vi "多路分流器测试.vi"() -> ()   [LabVIEW 2021]
uses:
  <vilib>/Utility/file.llb/Read Delimited Spreadsheet (DBL).vi
  <vilib>/Utility/file.llb/Write Delimited Spreadsheet (string).vi
  <instrlib>/Keithley 27XX/Keithley 27XX.lvlib
  <instrlib>/TDK-Lambda G Series/TDK-Lambda G Series.lvlib
  <instrlib>/Keithley DMM6500 DAQ6500 Series/Keithley DMM6500 DAQ6500 Series.lvlib
panel:
  out "报文数组":string[][](array[string])
  out "10帧平均总判定":bool
  out "判定 2":bool[](array[boolean])
  out "10帧平均误差":dbl[](array[numeric])
  in  "传感器缩放系数":dbl=2000.0 format="%#_13g"
  in  "产品类型":string
  in  "零漂2":dbl=0.01 format="%#_13g"
  in  "精度":dbl=0.005 format="%#_13g"
  out "误差":dbl[](array[numeric])
  out "解析电流":dbl[](array[numeric])
  out "判定":bool
  out "判定":bool[](array[boolean])
  in  "CAN卡类型选择":T1
  in  "ID":string
  in  "CAN通道in":u16[](array[numeric])=[81, 82, 83]
  in  "file path (dialog if empty)":path caption="文件路径 （空时为对话框）"
  out "延迟时间":dbl[](array[numeric])=[0.0, 20.0, 5.0, 5.0, 1.0, 0.1, 0.1, 0.1, 0.1, 0.1, 0.1]
  in  "2700":refnum<visa-resource-name>="GPIB0::16::INSTR"
  out "测试电流":dbl[](array[numeric])=[0.0, 50.0, 100.0, 150.0, 200.0, 250.0, 300.0, 350.0, 400.0, 500.0, 1000.0]
  out "实际电流":dbl[](array[numeric])
  # "数据文件在F:\\shunt"
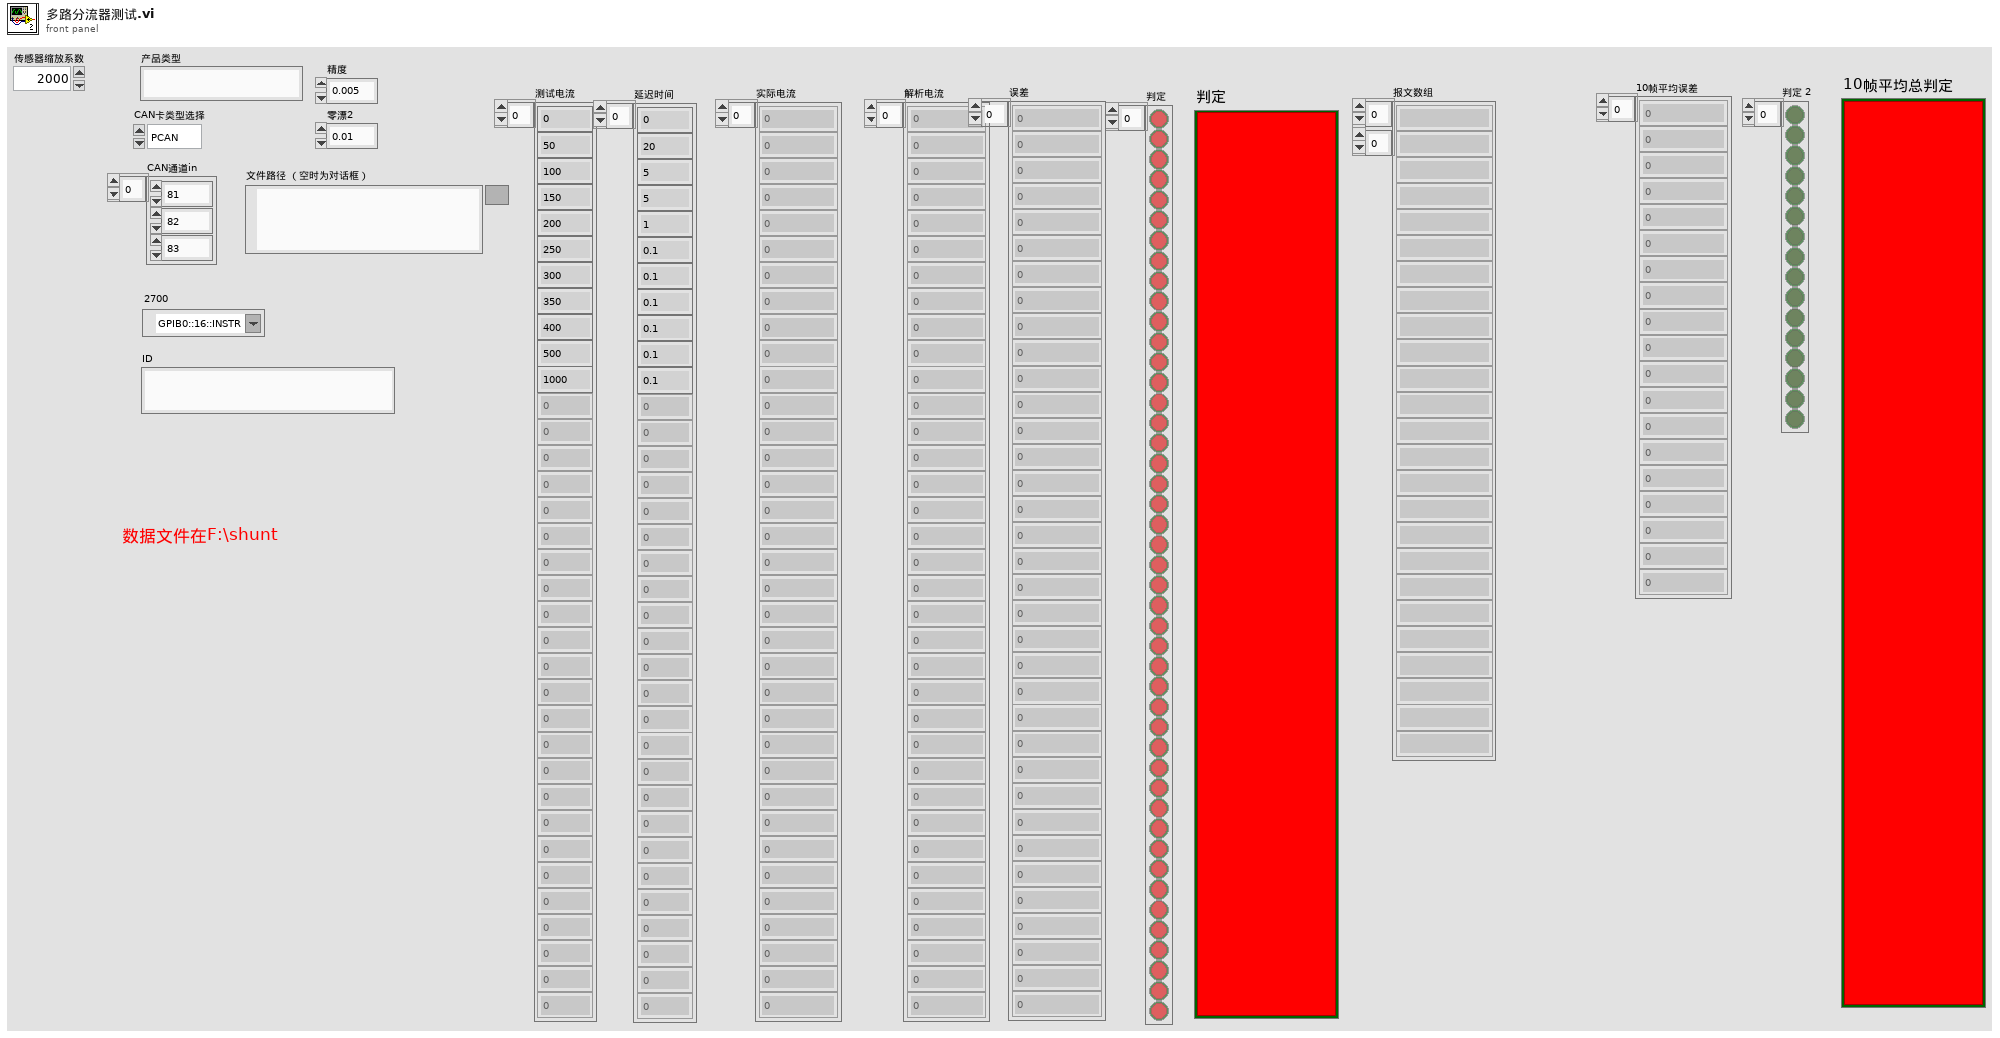
[diagram p1: front panel]
types:
  T1 = typedef "CAN type.ctl" = enum16{"PCAN", "PCANFD"}
  T2 = enum16{"open", "replace", "create", "open or create", "replace or create", "replace or create with confirmation"}
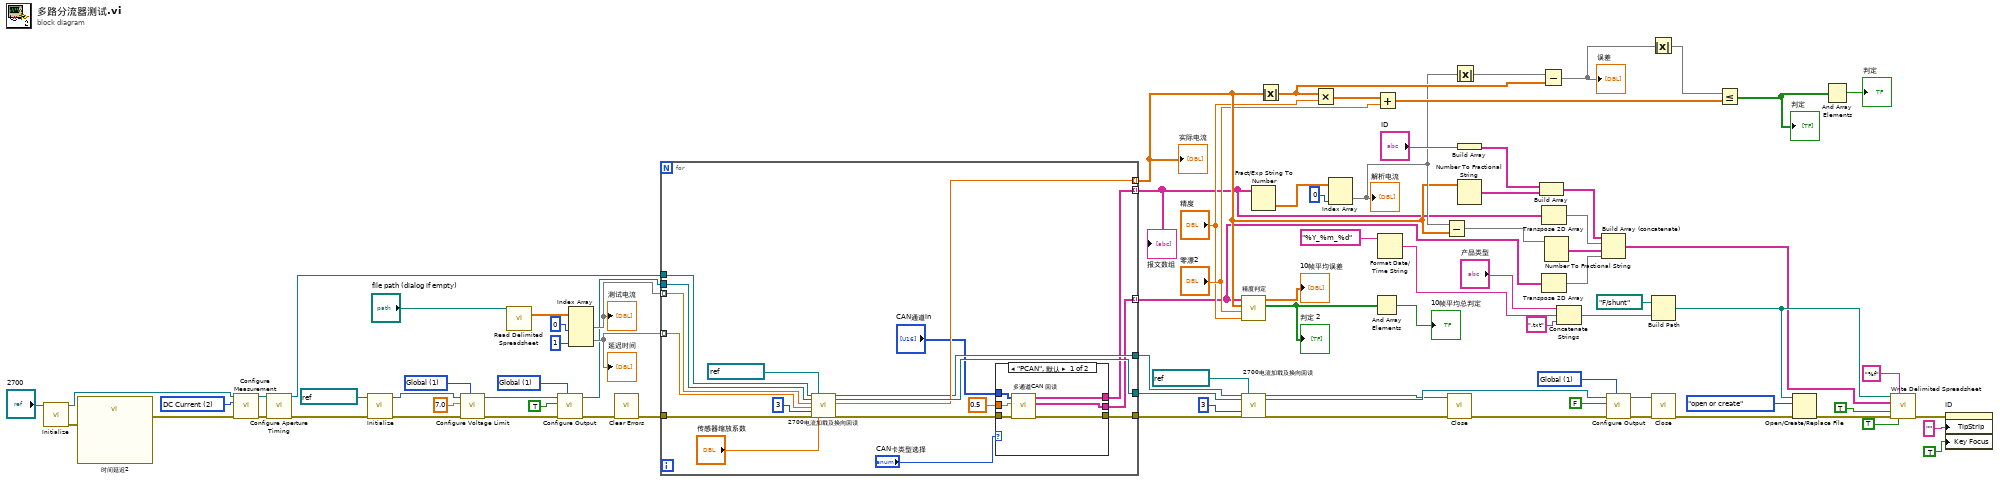
[diagram p0: block diagram]
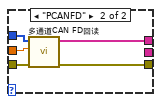
[diagram p2: hidden frame]
diagram:
  w39 = u16 2 items=["DC Voltage", "AC Voltage", "DC Current", "AC Current", "Resistance", "Four-Wire Resistance", "Temperature", "Frequency", "Period", "Continuity"] ("Function (0: DC Voltage)")
  w72 = u16 1 items=["Single", "Global"] ("Globalize (0: Single)")
  w74 = u16 1 items=["Single", "Global"] ("Globalize (0: Single)")
  w78 = u16 1 items=["Single", "Global"] ("Globalize (0: Single)")
  n1 = call <instrlib>:"Initialize.vi"("VISA resource name"="2700") -> ("VISA resource name out"=w41:refnum<visa-resource-name>, "error out"=w42:errorcluster)  [unwired: 13 in]
  n2 = call "时间延迟2"("error in (no error)"=w42) -> ("error out"=w40:errorcluster)  [unwired: 10 in]
  n3 = call <instrlib>:"Configure Measurement.vi"("VISA resource name"=w41, "Function (0: DC Voltage)"=w39, "error in (no error)"=w40) -> ("VISA resource name out"=w38:refnum<visa-resource-name>, "error out"=w37:errorcluster)  [unwired: 11 in]
  n4 = call <instrlib>:"Configure Aperture Timing.vi"("VISA resource name"=w38, "error in (no error)"=w37) -> ("VISA resource name out"=w32:refnum<visa-resource-name>, "error out"=w36:errorcluster)  [unwired: 12 in]
  n5 = call <instrlib>:"Initialize.vi"("error in (no error)"=w36, "VISA resource name"=refnum<visa-resource-name> "COM15") -> ("error out"=w79:errorcluster, "VISA resource name out"=w80:refnum<visa-resource-name>)  [unwired: 8 in]
  n6 = call <instrlib>:"Configure Voltage Limit.vi"("Globalize (0: Single)"=w78, "error in (no error)"=w79, "Voltage Limit (0V)"=7.0, "VISA resource name"=w80) -> ("error out"=w77:errorcluster, "VISA resource name out"=w76:refnum<visa-resource-name>)  [unwired: 6 in]
  n7 = call-poly <vilib>:"Read Delimited Spreadsheet.vi"("file path (dialog if empty)"="file path (dialog if empty)") -> ("all rows"=w55:dbl[][])  [unwired: 9 in, 5 out]
  n8 = call <instrlib>:"Configure Output.vi"("Globalize (0: Single)"=w74, "error in (no error)"=w77, "Enable Output (False)"=TRUE, "VISA resource name"=w76) -> ("error out"=w35:errorcluster, "VISA resource name out"=w33:refnum<visa-resource-name>)  [unwired: 6 in]
  n9 = Index Array(array=w55, index (col) #1=0 ("禁用的索引 (列)"), index (col) #2=1 ("索引 (列)")) -> (element #1=w52:dbl[], element #2=w51:dbl[])  [unwired: 2 in]
  "测试电流" <- w52
  "延迟时间" <- w51
  n10 = call <vilib>:"Clear Errors.vi"("error in (no error)"=w35) -> ("error out"=w34:errorcluster)  [unwired: 5 in, 1 out]
  n11 = for {
    tunnel: w33 -> [w94]
    tunnel: w34 -> [w102]
    tunnel: [w100] -> w83
    tunnel: [w88] -> w46
    tunnel: [w99] -> w8 mode=indexing
    tunnel: w52 -> [w98] mode=indexing
    tunnel: w51 -> [w96] mode=indexing
    tunnel: w32 -> [w95]
    tunnel: [w93] -> w50
    tunnel: [w87] -> w1 mode=indexing
    tunnel: [w85] -> w2 mode=indexing
    n12 = call "2700电流加载及换向回读.vi"("6510 in"=w95, "TDK in"=w94, "输入电流"=w98, "Delay Time (s)"=w96, "电源台数"=u8 3, "error in"=w102, "modbusin"=refnum<visa-resource-name> "COM12" ("VISA resource name"), "y"="传感器缩放系数") -> ("2700 out"=w93:refnum<visa-resource-name>, "TDK out"=w100:refnum<visa-resource-name>, "实际电流"=w99:dbl, "error out"=w91:errorcluster)  [unwired: 8 in]
    n13 = case shown="\"PCAN\", 默认" "CAN卡类型选择" {
      tunnel: w91 -> [w108 w111]
      tunnel: 0.5 ("Delay Time (s)") -> [w107 w112]
      tunnel: "CAN通道in" -> [w106 w113]
      tunnel: [w105 w110] -> w88
      tunnel: [w103 w109] -> w87
      tunnel: [w104 _] -> w85
      frame "PCAN", Default {
        n14 = call "多通道CAN 回读.vi"("错误输入（无错误）"=w108, "Delay Time (s)"=w107, "CAN通道in"=w106) -> ("错误输出"=w105:errorcluster, "10次平均"=w104:string[], "报文数组"=w103:string[])  [unwired: 6 in]
      }
      frame "PCANFD" {
        n15 = call "多通道CAN FD回读.vi"("错误输入（无错误）"=w111, "Delay Time (s)"=w112, "CAN通道in"=w113) -> ("错误输出"=w110:errorcluster, "报文数组"=w109:string[])  [unwired: 7 in]
      }
    }
  }
  "实际电流" <- w8
  "报文数组" <- w1
  n16 = call "精度判定.vi"("精度"="精度", "零飘"="零漂2", "实际电流"=w8, "报文数组"=w2) -> ("判定"=w3:bool[], "误差"=→"10帧平均误差":dbl[])  [unwired: 6 in]
  "判定 2" <- w3
  n17 = call "2700电流加载及换向回读.vi"("6510 in"=w50, "TDK in"=w83, "电源台数"=u8 3, "error in"=w46, "modbusin"=refnum<visa-resource-name> "COM12" ("VISA resource name")) -> ("2700 out"=w49:refnum<visa-resource-name>, "TDK out"=w71:refnum<visa-resource-name>, "error out"=w48:errorcluster)  [unwired: 11 in, 1 out]
  n18 = Fract/Exp String To Number(string=w1) -> (number=w26:dbl[][])  [unwired: 3 in, 1 out]
  n19 = Absolute Value(x=w8) -> (abs(x)=w23:dbl[])
  n20 = Multiply(x=w23, y="精度") -> (x*y=w22:dbl[])
  n21 = Index Array(array=w26, index (col)=0 ("禁用的索引 (列)")) -> (element=w13:dbl[])  [unwired: 1 in]
  "解析电流" <- w13
  n22 = And Array Elements(Boolean array=w3) -> (logical AND=→"10帧平均总判定":bool)
  n23 = Add(x=w22, y="零漂2") -> (x+y=w21:dbl[])
  n24 = Format Date/Time String(time format string (%c)="%Y_%m_%d" ("时间格式字符串(%c)")) -> (date/time string=w65:string)  [unwired: 2 in]
  n25 = Subtract(x=w13, y=w8) -> (x-y=w12:dbl[])
  n26 = call <instrlib>:"Close.vi"("error in (no error)"=w48, "VISA resource name"=w49) -> ("error out"=w47:errorcluster)  [unwired: 9 in]
  n27 = Absolute Value(x=w13) -> (abs(x)=w24:dbl[])
  n28 = Build Array("ID") -> (w31:string[])
  n29 = Number To Fractional String(number=w8) -> (F-format string=w30:string[])  [unwired: 3 in]
  n30 = Build Array(w31, w30) -> (w29:string[][])
  n31 = Subtract(x=w24, y=w23) -> (x-y=w15:dbl[])
  "误差" <- w15
  n32 = Transpose 2D Array(2D array=w1) -> (transposed array=w27:string[][])
  n33 = Transpose 2D Array(2D array=w2) -> (transposed array=w9:string[][])
  n34 = Number To Fractional String(number=w12) -> (F-format string=w11:string[])  [unwired: 3 in]
  n35 = Concatenate Strings("产品类型", w65, ".txt" ("字符串")) -> (w63:string)
  n36 = Build Array (concatenate)(w29, w27, w11, w9) -> (w28:string[][])
  n37 = call <instrlib>:"Configure Output.vi"("Globalize (0: Single)"=w72, "error in (no error)"=w47, "Enable Output (False)"=FALSE, "VISA resource name"=w71) -> ("error out"=w73:errorcluster, "VISA resource name out"=w70:refnum<visa-resource-name>)  [unwired: 6 in]
  n38 = Absolute Value(x=w15) -> (abs(x)=w14:dbl[])
  n39 = Build Path(base path=path "F:/shunt" ("file path (dialog if empty)"), name or relative path=w63) -> (appended path=w60:path)
  n40 = call <instrlib>:"Close.vi"("error in (no error)"=w73, "VISA resource name"=w70) -> ("error out"=w45:errorcluster)  [unwired: 9 in]
  n41 = Less Or Equal?(x=w14, y=w21) -> (x <= y?=w10:bool[])
  "判定" <- w10
  n42 = Open/Create/Replace File(file path (use dialog)=w60, error in=w45, operation (0:open)=T2."open or create" ("操作(0:open)")) -> (error out=w61:errorcluster)  [unwired: 3 in, 2 out]
  n43 = And Array Elements(Boolean array=w10) -> (logical AND=→"判定":bool)
  n44 = call-poly <vilib>:"Write Delimited Spreadsheet.vi"("file path (dialog if empty)"=w60, "format (%s)"="%f" ("format (%.3f)"), "2D data"=w28, "append to file? (new file:F)"=TRUE, "error in (no error)"=w61, "transpose? (no:F)"=TRUE) -> ("error out"=w19:errorcluster)  [unwired: 8 in, 1 out]
  n45 = property on="ID" class="Str"(error in=w19, "TipStrip"="" ("ID"), "Key Focus"=TRUE ("键选中")) -> ()  [unwired: 1 in, 2 out]
